vi "Examine Path.vi"(8 "error in":errorcluster caption="错误输入", 11 "Filename":string="MianData.xml") -> (0 "error out":errorcluster, 3 "Path":path)   [LabVIEW 2020]
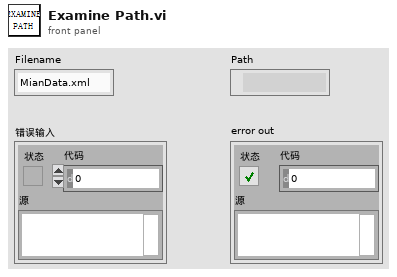
[diagram p1: front panel]
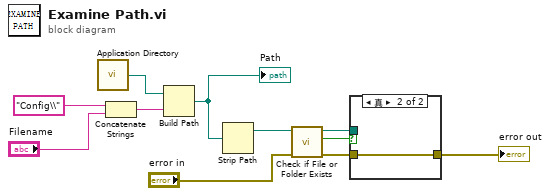
[diagram p0: block diagram]
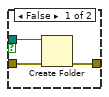
[diagram p2: hidden frame]
diagram:
  n1 = call <vilib>:"Application Directory.vi"() -> ("Application Directory"=w11:path)
  n2 = Concatenate Strings("Config\\" ("字符串"), "Filename") -> (w8:string)
  n3 = Build Path(base path=w11, name or relative path=w8) -> (appended path=w3:path)
  "Path" <- w3
  n4 = Strip Path(path=w3) -> (stripped path=w7:path)  [unwired: 1 out]
  n5 = call <vilib>:"Check if File or Folder Exists.vi"("error in (no error)"="error in", "path"=w7) -> ("error out"=w4:errorcluster, "file or folder exists?"=w6:bool, "dup path"=w5:path)  [unwired: 7 in]
  n6 = case shown="真" w6 {
    tunnel: w5 -> [w14 _]
    tunnel: w4 -> [w13 w15]
    tunnel: [w12 w15] -> w2
    frame False {
      n7 = Create Folder(path (use dialog)=w14, error in=w13) -> (error out=w12:errorcluster)  [unwired: 1 in, 2 out]
    }
    frame True {
    }
  }
  "error out" <- w2
